vi "scaninput.vi"(8 "error in (no error)":errorcluster, 11 "DMC1000B in":refnum<class "DMC1000B.lvclass">) -> (0 "error out":errorcluster, 3 "DMC1000B out":refnum<class "DMC1000B.lvclass">)   [LabVIEW 2019, in "DMC1000B.lvclass"]
uses:
  DMC1000B.lvclass
  LLB/DMC1000B/Dmc1000/Dmc1000.lvlib
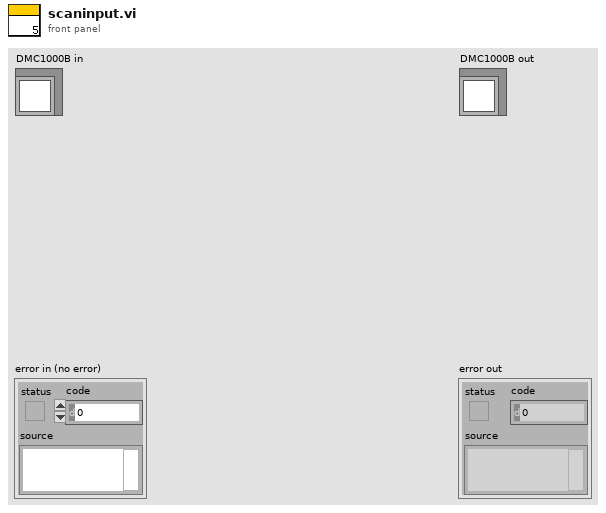
[diagram p1: front panel]
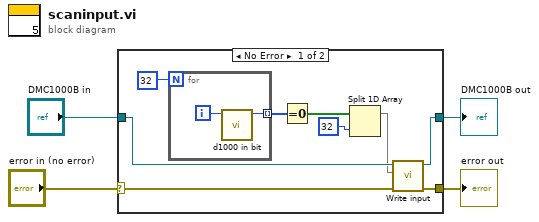
[diagram p0: block diagram]
diagram:
  n1 = case shown="No Error" "error in (no error)" {
    selector: "error in (no error)" -> [w5 w16]
    tunnel: "DMC1000B in" -> [w9 w17]
    tunnel: [w7 w17] -> w3
    tunnel: [w6 w16] -> w2
    frame No Error {
      n2 = for {
        N: 32 -> [_]
        tunnel: [w14] -> w12 mode=indexing
        i -> [w15]
        n3 = call "d1000 in bit.vi"("BitNo"=w15) -> ("function return"=w14:u32)  [unwired: 10 in]
      }
      n4 = Equal To 0?(x=w12) -> (x = 0?=w11:bool[])
      n5 = Split 1D Array(array=w11, index=32) -> (first subarray=w8:bool[])  [unwired: 1 out]
      n6 = call-dynamic "Write input.vi"("error in (no error)"=w5, "input"=w8, "IOCard in"=w9) -> ("error out"=w6:errorcluster, "IOCard out"=w7:refnum<class "DMC1000B.lvclass">)  [unwired: 7 in]
    }
    frame Error {
    }
  }
  "error out" <- w2
  "DMC1000B out" <- w3
